vi "E3640A Commands SA 2.vi"(0 "VISA session":refnum<visa-resource-name>="COM12", 7 "Command":u16(ring) items=["Output Off", "Output On", "Output?", "Voltage Range Low", "Voltage Range High", "Voltage Range?", "Apply 12V, 1.5A", "Apply?", "Voltage 12V", "Voltage?", "Current 1.5A", "Current?", "Measure Voltage", "Measure Current", "Set RS232", "Set Remote Mode", "Set Local Mode", "System Error?", "*IDN?", "*RST", "Instrument Sel?", "Instrument Sel Out 1", "Instrument Sel Out 2", "Display Mode VI", "Display Mode VV", "Display Mode II", "Voltage 10V", "Voltage 14V"], 11 "error in (no error)":errorcluster) -> (4 "VISA session out":refnum<visa-resource-name>, 6 "Response":string, 8 "Num Resp":dbl, 13 "Bytes at port":u8, 14 "Bytes Read":u8, 15 "error out":errorcluster)   [LabVIEW 2010]
uses:
  <vilib>/Instr/_visa.llb/VISA Configure Serial Port (Instr).vi
panel:
  in  "Serial Configuration":T1={"Baud Rate"=9600, "Parity"=0, "Data Bits"=8, "Stop Bits"=20, "Flow Control"=0} {"Flow Control" items=["None", "XON/XOFF", "RTS/CTS", "XON/XOFF & RTS/CTS", "DTR/DSR", "XON/XOFF & DTR/DSR"]; "Stop Bits" items=["1.0"=10, "1.5"=15, "2.0"=20]; "Data Bits" items=["7"=7, "8"=8]; "Parity" items=["None", "Odd", "Even", "Mark", "Space"]; "Baud Rate" items=["300"=300, "600"=600, "1200"=1200, "2400"=2400, "4800"=4800, "9600"=9600, "19200"=19200]}
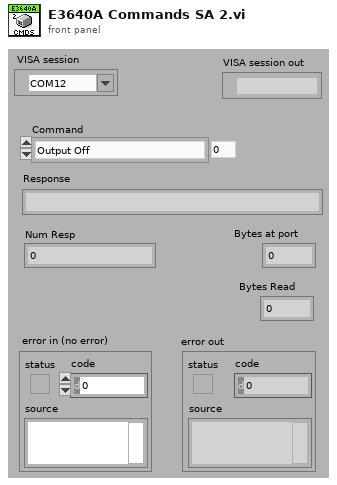
[diagram p1: front panel]
types:
  T1 = cluster{"Baud Rate":u32, "Parity":u16, "Data Bits":u16, "Stop Bits":u16, "Flow Control":u16}
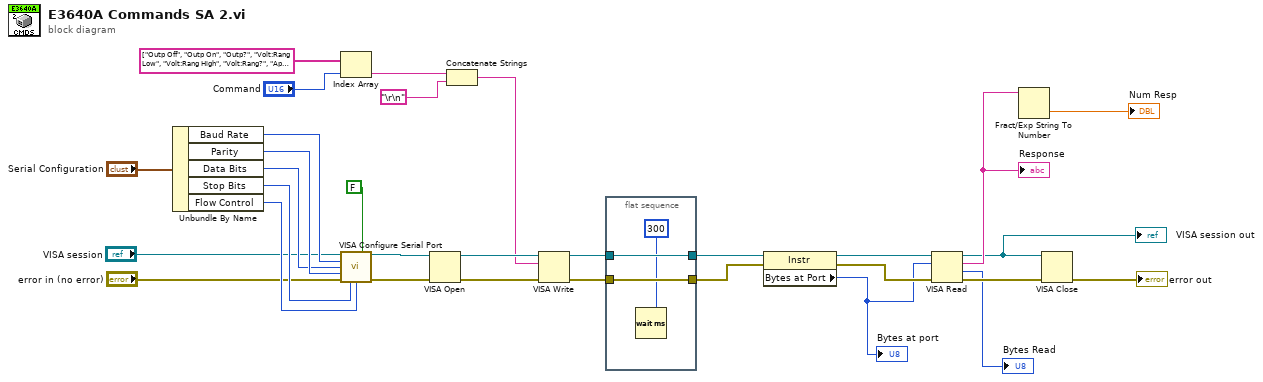
[diagram p0: block diagram]
diagram:
  n1 = Unbundle By Name("Serial Configuration") -> ("Baud Rate"=w30:u32, "Parity"=w29:u16, "Data Bits"=w28:u16, "Stop Bits"=w27:u16, "Flow Control"=w26:u16)
  n2 = Index Array(array=string[] ["Outp Off", "Outp On", "Outp?", "Volt:Rang Low", "Volt:Rang High", "Volt:Rang?", "Apply 12,1.5", "Apply?", "Volt 12", "Volt?", "Curr 1.5", "Curr?", "Meas:Volt?", "Meas:curr?", "Syst:Int RS232", "Syst:Rem", "Syst:Loc", "Syst:Err?", "*IDN?", "*RST", "INST:SEL?", "INST:SEL OUT1", "INST:SEL OUT2", "DISP:MODE VI", "DISP:MODE VV", "DISP:MODE II", "Volt 10", "Volt 14"], index="Command") -> (element=w2:string)
  n3 = call-poly "VISA Configure Serial Port"("VISA resource name"="VISA session", "Enable Termination\nChar (T)"=FALSE, "baud rate (9600)"=w30, "data bits (8)"=w28, "parity (0:none)"=w29, "error in (no error)"="error in (no error)", "stop bits (10: 1 bit)"=w27, "flow control (0:none)"=w26) -> ("VISA resource name out"=w22:refnum<visa-resource-name>, "error out"=w21:errorcluster)  [unwired: 6 in]
  n4 = VISA Open(error in (no error)=w21, VISA resource name=w22) -> (VISA resource name=w19:refnum<visa-resource-name>, error out=w20:errorcluster)  [unwired: 3 in]
  n5 = Concatenate Strings(w2, "\r\n") -> (w17:string)
  n6 = VISA Write(VISA resource name=w19, write buffer=w17, error in (no error)=w20) -> (VISA resource name out=w10:refnum<visa-resource-name>, error out=w9:errorcluster)  [unwired: 1 out]
  n7 = flat-sequence {
    tunnel: [w34] -> w7
    tunnel: w10 -> [w34]
    tunnel: [w33] -> w8
    tunnel: w9 -> [w33]
    frame #0 {
      n8 = Wait (ms)(milliseconds to wait=300) -> ()  [unwired: 1 out]
    }
  }
  n9 = property class="Instr"(reference=w7, error in=w8) -> (reference out=w13:refnum<visa-resource-name>, error out=w12:errorcluster, "Bytes at Port"=w11:u32)
  "Bytes at port" <- w11
  n10 = VISA Read(VISA resource name=w13, byte count=w11, error in (no error)=w12) -> (VISA resource name out=w1:refnum<visa-resource-name>, read buffer=w6:string, return count=→"Bytes Read":u32, error out=w15:errorcluster)
  "Response" <- w6
  "VISA session out" <- w1
  n11 = Fract/Exp String To Number(string=w6) -> (number=→"Num Resp":dbl)  [unwired: 3 in, 1 out]
  n12 = VISA Close(VISA resource name=w1, error in (no error)=w15) -> (error out=→"error out":errorcluster)
